vi "VCS Get Position Profile.vi"(8 "error in (no error)":errorcluster, 11 "axis in":cluster{"keyHandle":u32, "nodeId":u16}={"keyHandle"=0, "nodeId"=1}) -> (0 "error out":errorcluster, 2 "position profile":T1, 3 "axis out":cluster{"keyHandle":u32, "nodeId":u16}={"keyHandle"=0, "nodeId"=1})   [LabVIEW 2010]
doc: "<B>VCS Get Position Profile</B> returns the position profile parameters."
uses:
  Resources/EposCmd.dll
  Resources/EposCmd64.dll
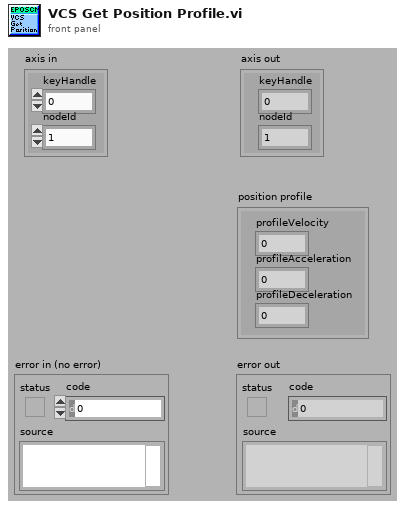
[diagram p1: front panel]
types:
  T1 = cluster{"profileVelocity":u32, "profileAcceleration":u32, "profileDeceleration":u32}
  T2 = cluster{"pProfileVelocity":u32, "pProfileAcceleration":u32, "pProfileDeceleration":u32}
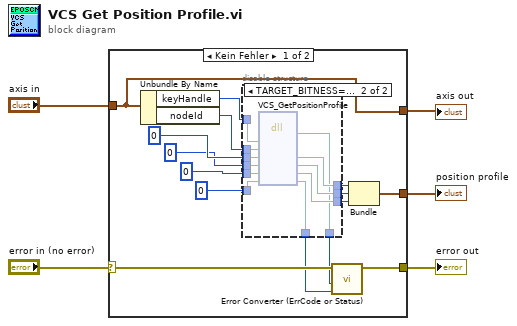
[diagram p0: block diagram]
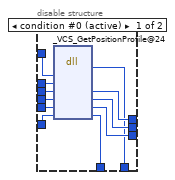
[diagram p2: hidden frame]
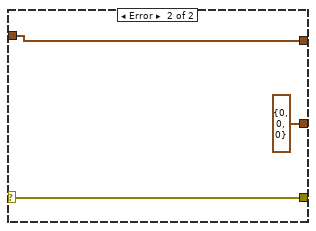
[diagram p3: hidden frame]
diagram:
  n1 = case shown="Kein Fehler" "error in (no error)" {
    selector: "error in (no error)" -> [w9 w45]
    tunnel: [w8 w45] -> w4
    tunnel: "axis in" -> [w10 w44]
    tunnel: [w11 T2 {"pProfileVelocity"=0, "pProfileAcceleration"=0, "pProfileDeceleration"=0}] -> w2
    tunnel: [w10 w44] -> w1
    frame No Error {
      n2 = Unbundle By Name(w10) -> ("keyHandle"=w20:u32, "nodeId"=w19:u16)
      n3 = disable-structure shown="TARGET_BITNESS==64" {
        disable-tunnel: w20 -> [w31 w42]
        disable-tunnel: w19 -> [w30 w41]
        disable-tunnel: u32 0 ("pProfileVelocity") -> [w29 w40]
        disable-tunnel: u32 0 ("pProfileAcceleration") -> [w28 w39]
        disable-tunnel: u32 0 ("pProfileDeceleration") -> [w27 w38]
        disable-tunnel: u32 0 ("pErrorCode") -> [w26 w37]
        disable-tunnel: [w25 w36] -> w14
        disable-tunnel: [w24 w35] -> w13
        disable-tunnel: [w23 w34] -> w12
        disable-tunnel: [w22 w33] -> w7
        disable-tunnel: [w21 w32] -> w6
        frame condition #0 (active) {
          n4 = dll-call lib="C:/Sources/LabView/maxon EPOS/Resources/EposCmd.*" fn="_VCS_GetPositionProfile@24"("KeyHandle"=w31, "NodeId"=w30, "pProfileVelocity"=w29, "pProfileAcceleration"=w28, "pProfileDeceleration"=w27, "pErrorCode"=w26) -> (w22:i32, "pProfileVelocity"=w25:u32, "pProfileAcceleration"=w24:u32, "pProfileDeceleration"=w23:u32, "pErrorCode"=w21:u32)  [unwired: 5 in, 2 out]
        }
        frame condition #1 {
          n5 = dll-call lib="C:/setup/Resources/EposCmd64.*" fn="VCS_GetPositionProfile" ("EposCmd.dll:_VCS_GetPositionProfile@24")("KeyHandle"=w42, "NodeId"=w41, "pProfileVelocity"=w40, "pProfileAcceleration"=w39, "pProfileDeceleration"=w38, "pErrorCode"=w37) -> ("Rückgabetyp"=w33:i32, "pProfileVelocity"=w36:u32, "pProfileAcceleration"=w35:u32, "pProfileDeceleration"=w34:u32, "pErrorCode"=w32:u32)  [unwired: 5 in, 2 out]
        }
      }
      n6 = call "Error Converter (ErrCode or Status).vi"("error code"=w6, "return type"=w7, "error in (no error)"=w9) -> ("error out"=w8:errorcluster)  [unwired: 7 in]
      n7 = Bundle("pProfileVelocity"=w14, "pProfileAcceleration"=w13, "pProfileDeceleration"=w12) -> (w11:T2)  [unwired: 1 in]
    }
    frame Error {
    }
  }
  "error out" <- w4
  "position profile" <- w2
  "axis out" <- w1
